vi "Saturation (DBL).vi"(2 "lower limit":dbl format="%.2f", 3 "upper limit":dbl format="%.2f", 4 "input point":dbl format="%.2f") -> (1 "output point":dbl format="%.2f")   [LabVIEW 2017, in "NI_AdvCtrl_nonlinear.lvlib"]
doc: "LabVIEW no longer supports this VI. You can obtain similar functionality by installing the LabVIEW Simulation Module.\n\nLimits the valid range of a signal. The output point is equal to the upper limit, if input point>upper limit. The output point is equal to the lower limit, if input point<lower limit. In all other cases it is output point=input point."
uses:
  <vilib>/addons/control/advanced/NI_AdvCtrl_nonlinear.lvlib
  <vilib>/addons/control/advanced/NI_AdvCtrl_continuous linear.lvlib
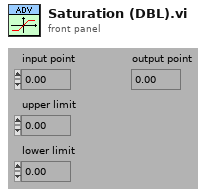
[diagram p1: front panel]
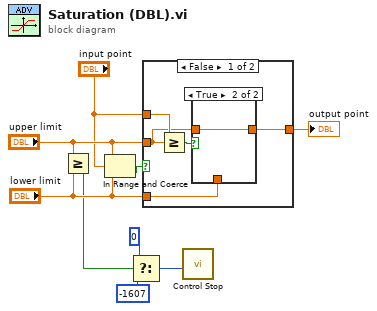
[diagram p0: block diagram]
diagram:
  n1 = Greater Or Equal?(x="upper limit", y="lower limit") -> (x >= y?=w2:bool)
  n2 = In Range and Coerce(upper limit="upper limit", x="input point", lower limit="lower limit") -> (In Range?=w5:bool)  [unwired: 1 out]
  n3 = Select(t=0, s=w2, f=-1607) -> (s? t:f=w1:i32)
  n4 = case shown="False" w5 {
    tunnel: "input point" -> [w14 w17]
    tunnel: [w11 w17] -> w7
    tunnel: "upper limit" -> [w12 _]
    tunnel: "lower limit" -> [w10 _]
    frame False {
      n5 = Greater Or Equal?(x=w14, y=w12) -> (x >= y?=w13:bool)
      n6 = case shown="True" w13 {
        tunnel: w12 -> [_ w16]
        tunnel: [w15 w16] -> w11
        tunnel: w10 -> [w15 _]
        frame False {
        }
        frame True {
        }
      }
    }
    frame True {
    }
  }
  "output point" <- w7
  n7 = call <vilib>:"Control Stop.vi"("error"=w1) -> ()  [unwired: 2 out]
